vi "File Path Generate and Write HCC Debug.vi"(7 "Use Day In Path":bool=TRUE, 8 "error in":errorcluster, 10 "Data Array":string[][](array[string]), 11 "base path":path) -> (0 "error out":errorcluster, 3 "new file path (Not A Path if cancelled)":path)   [LabVIEW 2009]
uses:
  <vilib>/Utility/file.llb/Write To Spreadsheet File (string).vi
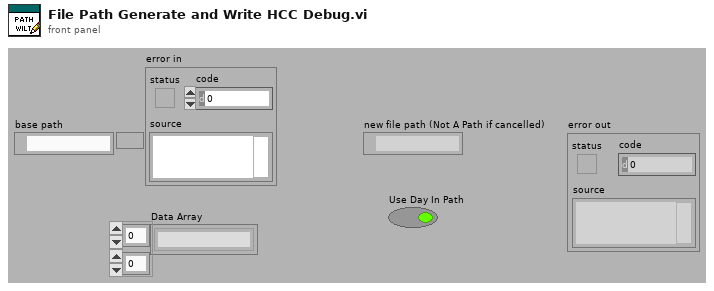
[diagram p1: front panel]
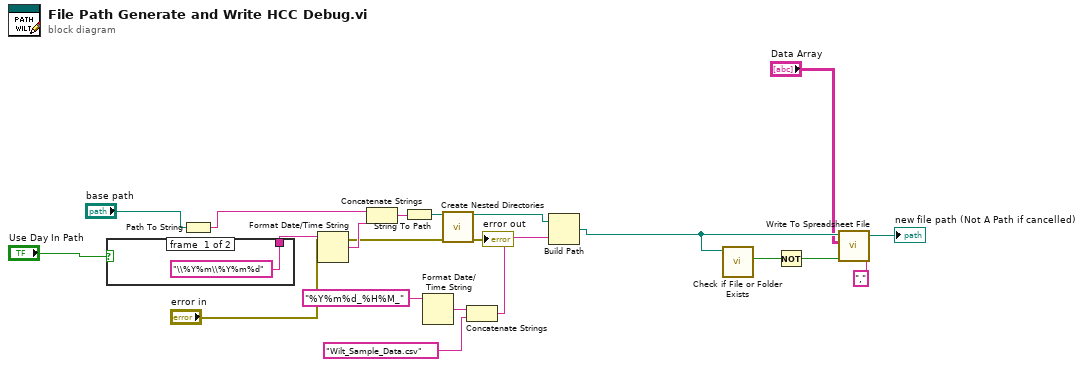
[diagram p0: block diagram]
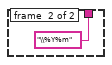
[diagram p2: hidden frame]
diagram:
  n1 = case shown="True" "Use Day In Path" {
    tunnel: ["\\%Y%m\\%Y%m%d" ("time format string (%c)") "\\%Y%m" ("time format string (%c)")] -> w20
    frame #0 {
    }
    frame #1 {
    }
  }
  n2 = Path To String(path="base path") -> (string=w11:string)
  n3 = Format Date/Time String(time format string (%c)=w20) -> (date/time string=w13:string)  [unwired: 2 out]
  n4 = Concatenate Strings(w11, w13) -> (w12:string)
  n5 = String To Path(string=w12) -> (path=w14:path)
  n6 = Format Date/Time String(time format string (%c)="%Y%m%d_%H%M_") -> (date/time string=w4:string)  [unwired: 2 out]
  n7 = call "Create Nested Directories.vi"("path to create"=w14, "error in"="error in") -> ("created path"=w16:path, "error out"=→"error out":errorcluster)  [unwired: 11 in, 1 out]
  n8 = Concatenate Strings(w4, "Wilt_Sample_Data.csv" ("string")) -> (w15:string)
  n9 = Build Path(base path=w16, name or relative path=w15) -> (appended path=w17:path)
  n10 = call <vilib>:"Check if File or Folder Exists.vi"("path"=w17) -> ("file or folder exists?"=w9:bool)  [unwired: 8 in, 2 out]
  n11 = Not(x=w9) -> (.not. x?=w18:bool)
  n12 = call-poly <vilib>:"Write To Spreadsheet File.vi"("delimiter (\\t)"="," ("delimiter (\\t)"), "append to file? (new file:F)"=w18, "2D data"="Data Array", "file path (dialog if empty)"=w17) -> ("new file path (Not A Path if cancelled)"=→"new file path (Not A Path if cancelled)":path)  [unwired: 4 in]
